vi "Path_Check if Relative.vi"(11 "Path":path) -> (3 "Relative Path?":bool)   [LabVIEW 2019, in "AutoMenuCreator.lvlib"]
uses:
  AutoMenuCreator.lvlib
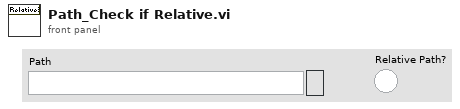
[diagram p1: front panel]
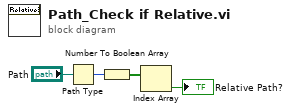
[diagram p0: block diagram]
diagram:
  n1 = Path Type(1:"Path") -> (0:w4:i16)
  n2 = Number To Boolean Array(number=w4) -> (Boolean array=w3:bool[])
  n3 = Index Array(array=w3) -> (element=→"Relative Path?":bool)  [unwired: 1 in]
